vi "save channels to stacked tiff series.vi"(8 "frame number in":i32, 9 "last frame":bool, 11 "image data in":dbl[][](array[numeric])) -> ()   [LabVIEW 2012]
uses:
  Custom Controls/file format type def.ctl
  GFG/GFGpathGet.vi
  GFG/GFGnumericGet.vi
  Libtiff3/libtiff3.llb/libtiff3.lvlib
  GFG/GFG library.lvlib
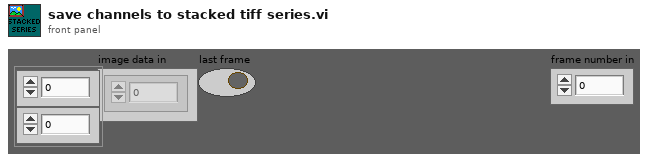
[diagram p1: front panel]
types:
  T1 = typedef "file format type def.ctl" = enum16{"16bit raw", "32bit raw", "16bit multi-tiff (interleave)", "16bit multi-tiff (separate)", "16bit multi-tiff (stacked)", "32bit multi-tiff (interleave)", "32bit multi-tiff (separate)", "32bit multi-tiff (stacked)", "16bit tiff series (interleave)", "16bit tiff series (separate)", "16bit tiff series (stacked)", "32bit tiff series (interleave)", "32bit tiff series (separate)", "32bit tiff series (stacked)"}
  T2 = cluster{"no..of.frames.to.acquire":dbl, "x.pixels":dbl, "y.pixels":dbl, "x.pixel.sz":dbl, "y.pixel.sz":dbl}
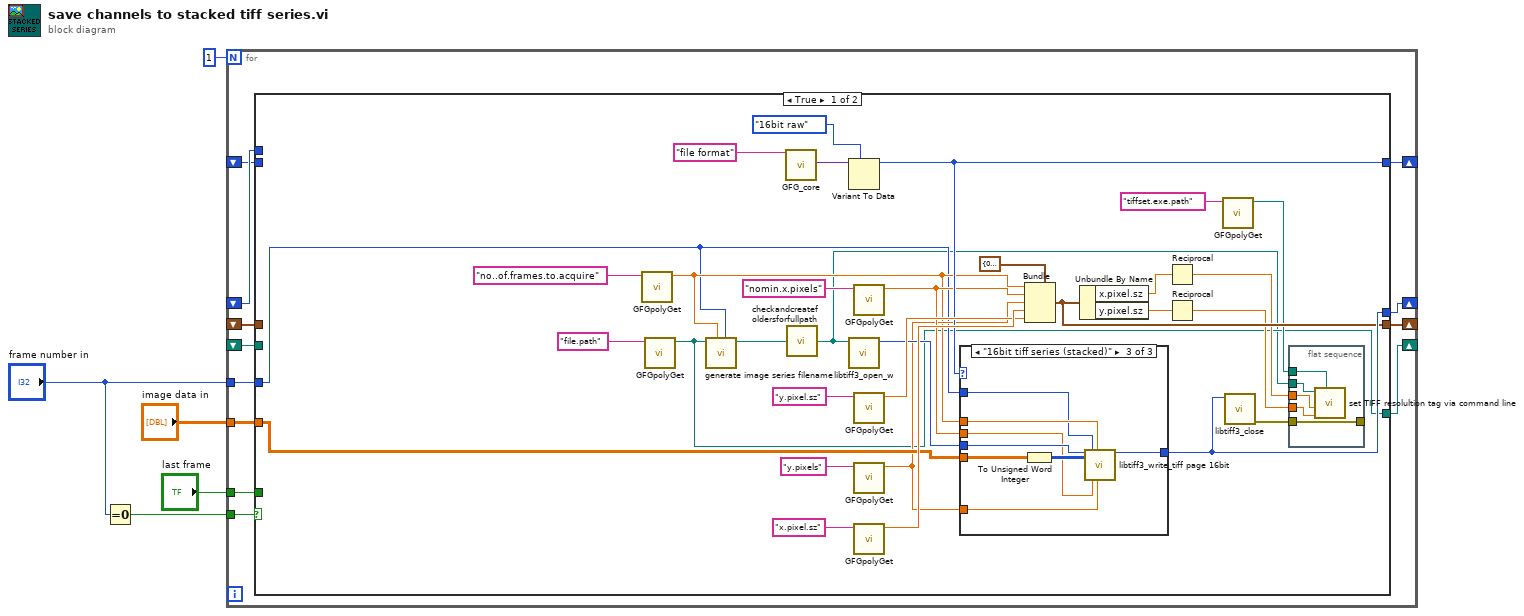
[diagram p0: block diagram]
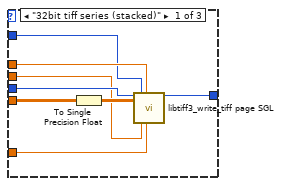
[diagram p2: hidden frame]
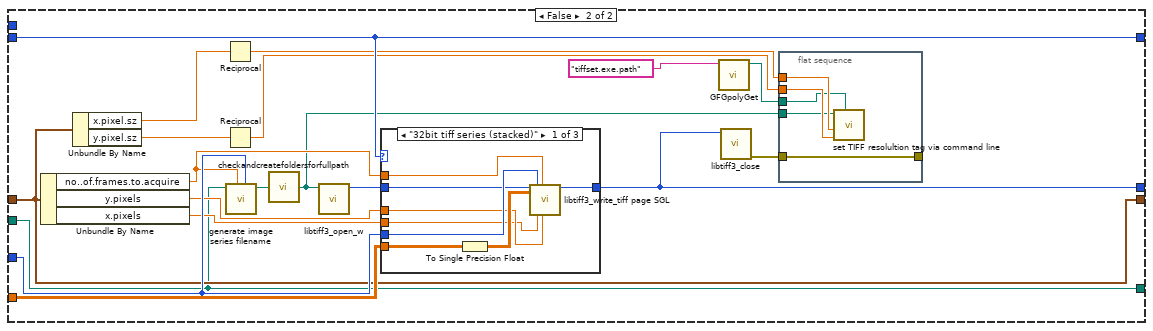
[diagram p4: hidden frame]
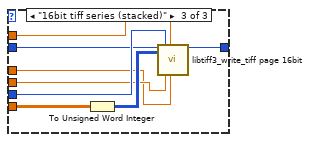
[diagram p6: hidden frame]
diagram:
  n1 = Equal To 0?(x="frame number in") -> (x = 0?=w4:bool)
  n2 = for {
    N: 1 -> [_]
    tunnel: w4 -> [w17]
    shift-right: [w16] -> _
    shift-left: _ -> [w15]
    tunnel: "image data in" -> [w14]
    shift-right: [w13] -> _
    shift-left: _ -> [w12]
    shift-right: [w11] -> _
    shift-left: _ -> [w10]
    shift-right: [w9] -> _
    shift-left: _ -> [w8]
    tunnel: "last frame" -> [w7]
    tunnel: "frame number in" -> [w6]
    n3 = case shown="True" w17 {
      tunnel: w12 -> [_ w84]
      tunnel: [w28 w80] -> w16
      tunnel: w15 -> [_ _]
      tunnel: w14 -> [w35 w86]
      tunnel: [w36 w84] -> w13
      tunnel: [w27 w81] -> w11
      tunnel: w10 -> [_ w81]
      tunnel: [w19 w72] -> w9
      tunnel: w8 -> [_ w72]
      tunnel: w7 -> [_ _]
      tunnel: w6 -> [w29 w87]
      frame True {
        n4 = call-poly "GFGpolyGet.vi"("Variable Name in"="no..of.frames.to.acquire") -> ("Numeric"=w30:dbl)  [unwired: 9 in, 1 out]
        n5 = call-poly "GFGpolyGet.vi"("Variable Name in"="file.path") -> ("Path"=w19:path)  [unwired: 9 in, 1 out]
        n6 = call "generate image series filename.vi"("frame number in"=w29, "no..of.frames.to.acquire"=w30, "Path IN"=w19) -> ("appended path"=w31:path)  [unwired: 8 in]
        n7 = call "GFG_core.vi"("Variable Name in"="file format") -> ("Variant Out"=w47:variant)  [unwired: 12 in, 6 out]
        n8 = call "checkandcreatefoldersforfullpath.vi"("Path IN"=w31) -> ("Path OUT"=w18:path)  [unwired: 4 in]
        n9 = Variant To Data(type=file_format_type_def."16bit raw" ("file format"), Variant=w47) -> (data=w36:T1)  [unwired: 1 in, 1 out]
        n10 = call "libtiff3_open_w.vi"("Input path"=w18) -> ("handle"=w34:i32)  [unwired: 9 in, 1 out]
        n11 = call-poly "GFGpolyGet.vi"("Variable Name in"="nomin.x.pixels" ("Tag in")) -> ("Numeric"=w33:dbl)  [unwired: 9 in, 1 out]
        n12 = call-poly "GFGpolyGet.vi"("Variable Name in"="y.pixel.sz" ("Tag in")) -> ("Numeric"=w38:dbl)  [unwired: 9 in, 1 out]
        n13 = call-poly "GFGpolyGet.vi"("Variable Name in"="y.pixels" ("Tag in")) -> ("Numeric"=w32:dbl)  [unwired: 9 in, 1 out]
        n14 = call-poly "GFGpolyGet.vi"("Variable Name in"="x.pixel.sz" ("Tag in")) -> ("Numeric"=w39:dbl)  [unwired: 9 in, 1 out]
        n15 = case shown="\"16bit tiff series (stacked)\"" w36 {
          tunnel: w35 -> [w57 _ w67]
          tunnel: w34 -> [w58 w62 w68]
          tunnel: w29 -> [w59 _ w69]
          tunnel: w30 -> [w60 _ w70]
          tunnel: [w61 w62 w63] -> w28
          tunnel: w33 -> [w54 _ w65]
          tunnel: w32 -> [w55 _ w64]
          frame "32bit tiff series (stacked)" {
            n16 = To Single Precision Float(number=w57) -> (single precision float=w56:sgl[][])
            n17 = call "libtiff3_write_tiff page SGL.vi"("Handle"=w58, "Image Pixels (Float)"=w56, "page"=w59, "x.pixels"=w54, "totalpages"=w60, "y.pixels"=w55) -> ("Handle out"=w61:i32)  [unwired: 12 in, 1 out]
          }
          frame Default {
          }
          frame "16bit tiff series (stacked)" {
            n18 = To Unsigned Word Integer(number=w67) -> (unsigned 16bit integer=w66:u16[][])
            n19 = call "libtiff3_write_tiff page 16bit.vi"("Handle"=w68, "Image Pixels (U16)"=w66, "page"=w69, "x.pixels"=w65, "totalpages"=w70, "y.pixels"=w64) -> ("Handle out"=w63:i32)  [unwired: 12 in, 1 out]
          }
        }
        n20 = Bundle(cluster=T2 {"no..of.frames.to.acquire"=0.0, "x.pixels"=0.0, "y.pixels"=0.0, "x.pixel.sz"=0.0, "y.pixel.sz"=0.0} ("output cluster"), "no..of.frames.to.acquire"=w30, "x.pixels"=w33, "y.pixels"=w32, "x.pixel.sz"=w39, "y.pixel.sz"=w38) -> (w27:T2)
        n21 = Unbundle By Name(w27) -> ("x.pixel.sz"=w22:dbl, "y.pixel.sz"=w23:dbl)
        n22 = Reciprocal(x=w22) -> (1/x=w24:dbl)
        n23 = Reciprocal(x=w23) -> (1/x=w25:dbl)
        n24 = call-poly "GFGpolyGet.vi"("Variable Name in"="tiffset.exe.path") -> ("Path"=w20:path)  [unwired: 9 in, 1 out]
        n25 = call "libtiff3_close.vi"("Handle"=w28) -> ("error out"=w26:errorcluster)  [unwired: 9 in]
        n26 = flat-sequence {
          tunnel: w26 -> [w51]
          tunnel: w24 -> [w53]
          tunnel: w25 -> [w52]
          tunnel: [w51] -> _
          tunnel: w20 -> [w50]
          tunnel: w18 -> [w49]
          frame #0 {
            n27 = call "set TIFF resolultion tag via command line.vi"("tiffset.exe file path"=w50, "y pixels per m"=w52, "x pixels per m"=w53, "TIFF file path"=w49) -> ()  [unwired: 8 in]
          }
        }
      }
      frame False {
        n28 = Unbundle By Name(w81) -> ("no..of.frames.to.acquire"=w85:dbl, "y.pixels"=w83:dbl, "x.pixels"=w82:dbl)
        n29 = Unbundle By Name(w81) -> ("x.pixel.sz"=w75:dbl, "y.pixel.sz"=w76:dbl)
        n30 = Reciprocal(x=w75) -> (1/x=w77:dbl)
        n31 = Reciprocal(x=w76) -> (1/x=w78:dbl)
        n32 = call "generate image series filename.vi"("frame number in"=w87, "no..of.frames.to.acquire"=w85, "Path IN"=w72) -> ("appended path"=w88:path)  [unwired: 8 in]
        n33 = call "checkandcreatefoldersforfullpath.vi"("Path IN"=w88) -> ("Path OUT"=w71:path)  [unwired: 4 in]
        n34 = call "libtiff3_open_w.vi"("Input path"=w71) -> ("handle"=w89:i32)  [unwired: 9 in, 1 out]
        n35 = case shown="\"32bit tiff series (stacked)\"" w84 {
          tunnel: w86 -> [w98 _ w108]
          tunnel: w89 -> [w99 w103 w109]
          tunnel: w87 -> [w100 _ w110]
          tunnel: w85 -> [w101 _ w111]
          tunnel: [w102 w103 w104] -> w80
          tunnel: w82 -> [w95 _ w106]
          tunnel: w83 -> [w96 _ w105]
          frame "32bit tiff series (stacked)" {
            n36 = To Single Precision Float(number=w98) -> (single precision float=w97:sgl[][])
            n37 = call "libtiff3_write_tiff page SGL.vi"("Handle"=w99, "Image Pixels (Float)"=w97, "page"=w100, "x.pixels"=w95, "totalpages"=w101, "y.pixels"=w96) -> ("Handle out"=w102:i32)  [unwired: 12 in, 1 out]
          }
          frame Default {
          }
          frame "16bit tiff series (stacked)" {
            n38 = To Unsigned Word Integer(number=w108) -> (unsigned 16bit integer=w107:u16[][])
            n39 = call "libtiff3_write_tiff page 16bit.vi"("Handle"=w109, "Image Pixels (U16)"=w107, "page"=w110, "x.pixels"=w106, "totalpages"=w111, "y.pixels"=w105) -> ("Handle out"=w104:i32)  [unwired: 12 in, 1 out]
          }
        }
        n40 = call-poly "GFGpolyGet.vi"("Variable Name in"="tiffset.exe.path") -> ("Path"=w73:path)  [unwired: 9 in, 1 out]
        n41 = call "libtiff3_close.vi"("Handle"=w80) -> ("error out"=w79:errorcluster)  [unwired: 9 in]
        n42 = flat-sequence {
          tunnel: w79 -> [w92]
          tunnel: w77 -> [w94]
          tunnel: w78 -> [w93]
          tunnel: [w92] -> _
          tunnel: w73 -> [w91]
          tunnel: w71 -> [w90]
          frame #0 {
            n43 = call "set TIFF resolultion tag via command line.vi"("tiffset.exe file path"=w91, "y pixels per m"=w93, "x pixels per m"=w94, "TIFF file path"=w90) -> ()  [unwired: 8 in]
          }
        }
      }
    }
  }
